vi "DTS-C.vi"() -> ()   [LabVIEW 2020]
uses:
  <vilib>/Utility/error.llb/DialogType.ctl
panel:
  in  "정지 버튼":bool
  out "XY Graph 2":cluster{"Y":dbl[], "Y":dbl[]}[](graph) caption="XY 그래프"
  out "대기중":bool
  out "XY Graph":cluster{"Y":dbl[], "Y":dbl[]}[](graph) caption="XY 그래프"
  out "안티스톡스":bool
  in  "안티 스톡스 측정 데이터 경로":path
  out "스톡스":bool
  in  "스톡스 측정 데이터 경로":path
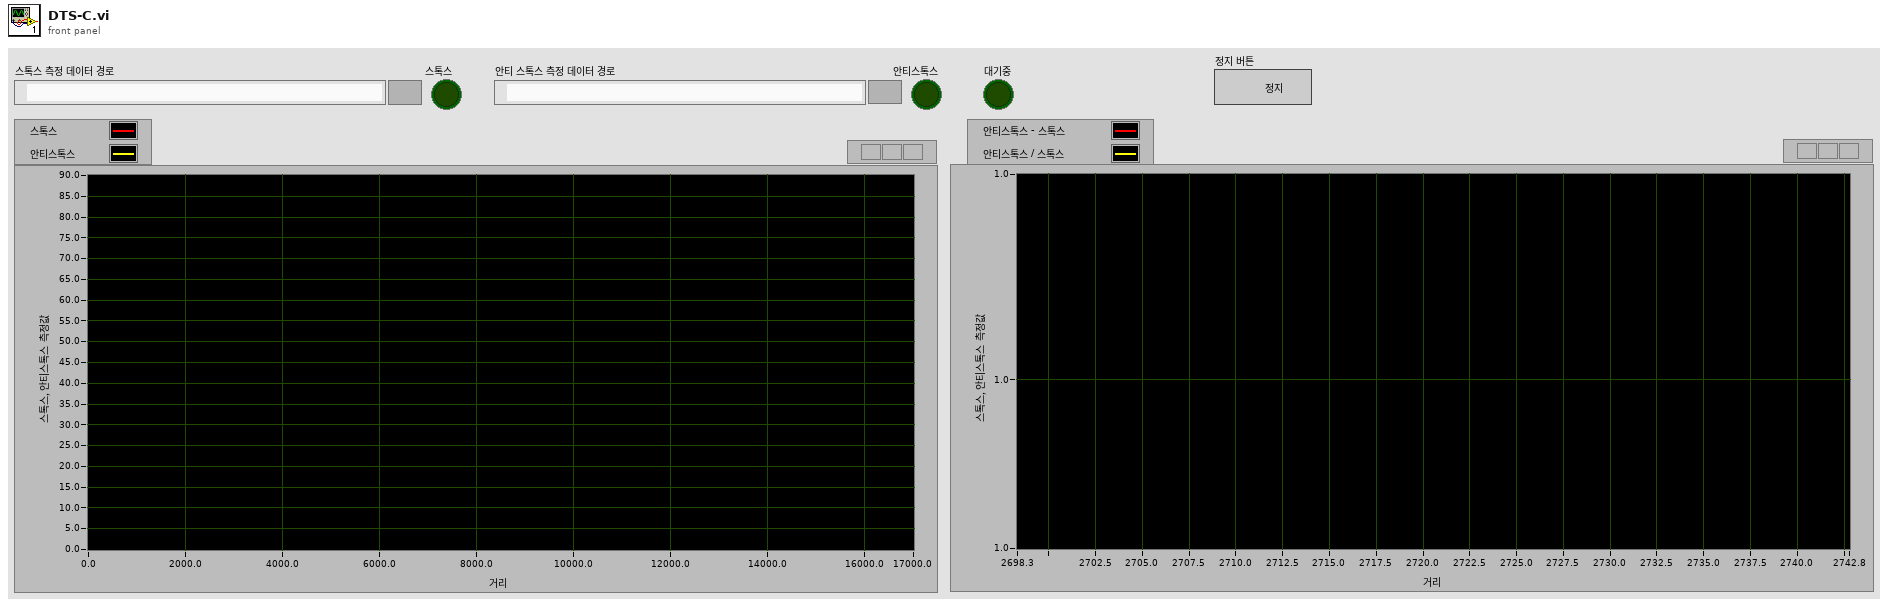
[diagram p1: front panel]
types:
  T1 = typedef "DialogType.ctl" = u16
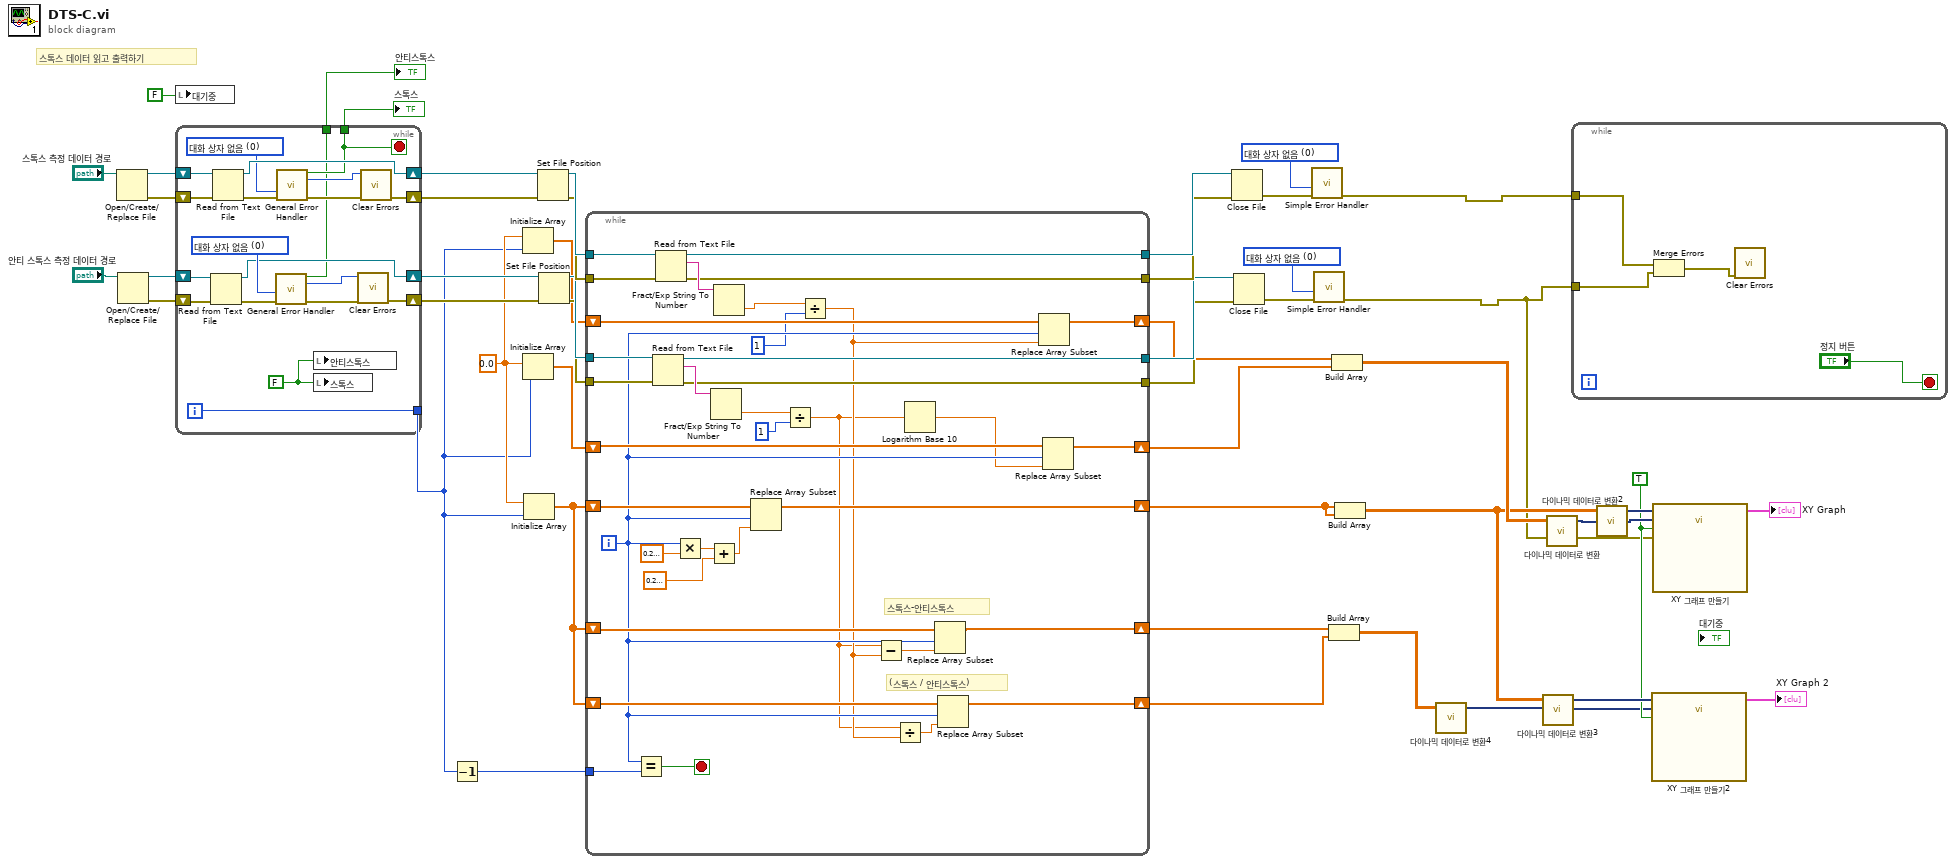
[diagram p0: block diagram]
diagram:
  w7 = TRUE ("Reset")
  w25 = T1 0 items=["대화 상자 없음", "확인 메시지", "메시지 지속 또는 정지", "확인 메시지 + 경고", "지속/정지 + 경고"] ("type of dialog (OK msg:1)")
  w37 = T1 0 items=["대화 상자 없음", "확인 메시지", "메시지 지속 또는 정지", "확인 메시지 + 경고", "지속/정지 + 경고"] ("type of dialog (OK msg:1)")
  w19 = 0.0 ("원소")
  # "스톡스 데이터 읽고 출력하기"
  n1 = Open/Create/Replace File(file path (use dialog)="스톡스 측정 데이터 경로") -> (refnum out=w46:refnum<file>, error out=w45:errorcluster)  [unwired: 5 in, 1 out]
  n2 = Open/Create/Replace File(file path (use dialog)="안티 스톡스 측정 데이터 경로") -> (refnum out=w32:refnum<file>, error out=w31:errorcluster)  [unwired: 5 in, 1 out]
  n3 = local write "대기중"(FALSE) -> ()
  n4 = while {
    shift-right: [w62] -> w42
    shift-left: w46 -> [w68]
    shift-right: [w63] -> w41
    shift-left: w45 -> [w67]
    tunnel: [w65] -> w18
    tunnel: [w59] -> w36
    shift-right: [w51] -> w29
    shift-left: w32 -> [w56]
    shift-right: [w52] -> w28
    shift-left: w31 -> [w55]
    tunnel: [w50] -> w30
    i -> [w65]
    stop <- w59 stop-if-true
    w57 = T1 0 items=["대화 상자 없음", "확인 메시지", "메시지 지속 또는 정지", "확인 메시지 + 경고", "지속/정지 + 경고"] ("type of dialog (OK msg:1)")
    w49 = FALSE
    w61 = T1 0 items=["대화 상자 없음", "확인 메시지", "메시지 지속 또는 정지", "확인 메시지 + 경고", "지속/정지 + 경고"] ("type of dialog (OK msg:1)")
    n5 = Read from Text File(file (use dialog)=w56, error in=w55) -> (refnum out=w51:refnum<file>, error out=w54:errorcluster)  [unwired: 2 in, 2 out]
    n6 = Read from Text File(file (use dialog)=w68, error in=w67) -> (refnum out=w62:refnum<file>, error out=w64:errorcluster)  [unwired: 2 in, 2 out]
    n7 = call <vilib>:"General Error Handler.vi"("type of dialog (OK msg:1)"=w57, "error in (no error)"=w54) -> ("error?"=w50:bool, "code out"=w58:i32, "error out"=w53:errorcluster)  [unwired: 9 in, 2 out]
    n8 = call <vilib>:"General Error Handler.vi"("type of dialog (OK msg:1)"=w61, "error in (no error)"=w64) -> ("error?"=w59:bool, "code out"=w66:i32, "error out"=w60:errorcluster)  [unwired: 9 in, 2 out]
    n9 = local write "안티스톡스"(w49) -> ()
    n10 = local write "스톡스"(w49) -> ()
    n11 = call <vilib>:"Clear Errors.vi"("error in (no error)"=w53, "specific error code to clear (0: all)"=w58) -> ("error out"=w52:errorcluster)  [unwired: 4 in, 1 out]
    n12 = call <vilib>:"Clear Errors.vi"("error in (no error)"=w60, "specific error code to clear (0: all)"=w66) -> ("error out"=w63:errorcluster)  [unwired: 4 in, 1 out]
  }
  "스톡스" <- w36
  "안티스톡스" <- w30
  n13 = Decrement(x=w18) -> (x-1=w34:i32)
  n14 = Initialize Array(w19, w18) -> (w17:dbl[])
  n15 = Initialize Array(w19, w18) -> (w47:dbl[])
  n16 = Initialize Array(w19, w18) -> (w21:dbl[])
  n17 = Set File Position(refnum=w42, error in=w41) -> (refnum out=w40:refnum<file>, error out=w39:errorcluster)  [unwired: 2 in]
  n18 = Set File Position(refnum=w29, error in=w28) -> (refnum out=w27:refnum<file>, error out=w23:errorcluster)  [unwired: 2 in]
  n19 = while {
    tunnel: w40 -> [w104]
    tunnel: w39 -> [w103]
    shift-right: [w77] -> w11
    shift-left: w47 -> [w78]
    tunnel: [w98] -> w44
    tunnel: [w97] -> w43
    shift-right: [w94] -> w16
    shift-left: w21 -> [w95]
    tunnel: w34 -> [w92]
    tunnel: w27 -> [w90]
    tunnel: [w89] -> w24
    tunnel: w23 -> [w88]
    tunnel: [w87] -> w22
    shift-right: [w85] -> w6
    shift-left: w21 -> [w84]
    shift-right: [w82] -> w5
    shift-left: w21 -> [w83]
    shift-right: [w79] -> w12
    shift-left: w17 -> [w80]
    i -> [w76]
    stop <- w93 stop-if-true
    # "(스톡스 / 안티스톡스)"
    # "스톡스-안티스톡스"
    n20 = Equal?(x=w76, y=w92) -> (x = y?=w93:bool)
    n21 = Read from Text File(file (use dialog)=w90, error in=w88) -> (refnum out=w89:refnum<file>, text=w91:string, error out=w87:errorcluster)  [unwired: 2 in, 1 out]
    n22 = Read from Text File(file (use dialog)=w104, error in=w103) -> (refnum out=w98:refnum<file>, text=w102:string, error out=w97:errorcluster)  [unwired: 2 in, 1 out]
    n23 = Multiply(x=w76, y=sgl 0.2) -> (x*y=w100:sgl)
    n24 = Add(x=w100, y=sgl 0.2) -> (x+y=w96:sgl)
    n25 = Fract/Exp String To Number(string=w91) -> (number=w75:dbl)  [unwired: 3 in, 1 out]
    n26 = Fract/Exp String To Number(string=w102) -> (number=w74:dbl)  [unwired: 3 in, 1 out]
    n27 = Replace Array Subset(array=w95, new element=w96, index=w76) -> (w94:dbl[])
    n28 = Divide(x=w75, y=u8 1 ("AS Gain")) -> (x/y=w69:dbl)
    n29 = Divide(x=w74, y=u8 1 ("S Gain")) -> (x/y=w70:dbl)
    n30 = Subtract(x=w69, y=w70) -> (x-y=w86:dbl)
    n31 = Divide(x=w69, y=w70) -> (x/y=w81:dbl)
    n32 = Logarithm Base 10(1:w69) -> (0:w71:dbl)
    n33 = Replace Array Subset(array=w84, new element=w86, index=w76) -> (w85:dbl[])
    n34 = Replace Array Subset(array=w83, new element=w81, index=w76) -> (w82:dbl[])
    n35 = Replace Array Subset(array=w80, new element=w70, index=w76) -> (w79:dbl[])
    n36 = Replace Array Subset(array=w78, new element=w71, index=w76) -> (w77:dbl[])
  }
  n37 = Close File(refnum=w44, error in=w43) -> (error out=w38:errorcluster)  [unwired: 1 out]
  n38 = Close File(refnum=w24, error in=w22) -> (error out=w26:errorcluster)  [unwired: 1 out]
  n39 = call <vilib>:"Simple Error Handler.vi"("type of dialog (OK msg:1)"=w37, "error in (no error)"=w38) -> ("error out"=w2:errorcluster)  [unwired: 3 in, 4 out]
  n40 = call <vilib>:"Simple Error Handler.vi"("type of dialog (OK msg:1)"=w25, "error in (no error)"=w26) -> ("error out"=w1:errorcluster)  [unwired: 3 in, 4 out]
  n41 = Build Array(w6, w5) -> (w4:dbl[][])
  n42 = Build Array(w12, w11) -> (w20:dbl[][])
  n43 = Build Array(w16, w16) -> (w9:dbl[][])
  n44 = call "다이나믹 데이터로 변환4"("2D Array"=w4) -> ("Dynamic Data Type"=w3:dynamicdata)  [unwired: 3 in]
  n45 = call "다이나믹 데이터로 변환3"("2D Array"=w9) -> ("Dynamic Data Type"=w8:dynamicdata)  [unwired: 3 in]
  n46 = call "다이나믹 데이터로 변환"("2D Array"=w20) -> ("Dynamic Data Type"=w13:dynamicdata)  [unwired: 3 in]
  n47 = while {
    tunnel: w2 -> [w107]
    tunnel: w1 -> [w106]
    stop <- "정지 버튼" stop-if-true
    n48 = Merge Errors(w107, w106) -> (w105:errorcluster)
    n49 = call <vilib>:"Clear Errors.vi"("error in (no error)"=w105) -> ()  [unwired: 5 in, 2 out]
  }
  n50 = call "다이나믹 데이터로 변환2"("2D Array"=w9) -> ("Dynamic Data Type"=w14:dynamicdata)  [unwired: 3 in]
  n51 = call "XY 그래프 만들기2"("Reset"=w7, "Y Input"=w3, "X Input"=w8) -> ("XY Graph"=→"XY Graph 2":cluster{"X":dbl[], "Y":dbl[]}[])  [unwired: 7 in, 1 out]
  n52 = call "XY 그래프 만들기"("error in (no error)"=w1, "Reset"=w7, "Y Input"=w13, "X Input"=w14) -> ("XY Graph"=→"XY Graph":cluster{"X":dbl[], "Y":dbl[]}[])  [unwired: 6 in, 1 out]
